vi "Compute Y's for equidistant Xn's.vi"(2 "Spline(T)":bool=TRUE, 3 "N":i16, 4 "Y":dbl[](array[numeric]) format="%.2e", 5 "X":dbl[](array[numeric]) format="%.2e") -> (0 "Yequi":dbl[](array[numeric]) format="%.2e", 1 "Xequi":dbl[](array[numeric]) format="%.2e")   [LabVIEW 2016]
doc: "Erzeugt zu einer XY-Meßkurve mit nicht \näquidistanten X-Werten eine zu \näquidistanten Werten. Die Größe N\nder neuen X- und Y-Arrays kann \ngrößer sein als die des Original X-Arrays.\nSpline gibt an, ob Spline- oder lineare\nInterpolation benutzt wird."
uses:
  <vilib>/Analysis/NI_AALPro.lvlib
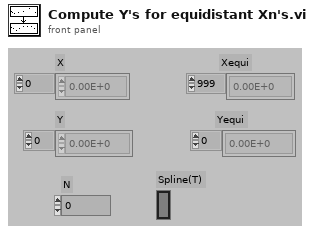
[diagram p1: front panel]
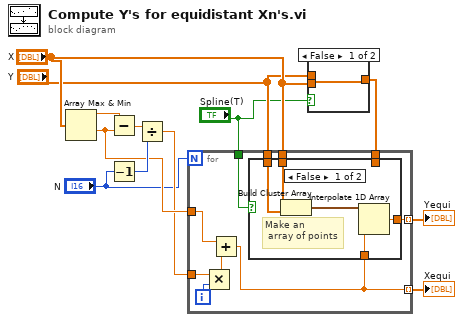
[diagram p0: block diagram]
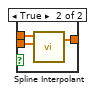
[diagram p2: hidden frame]
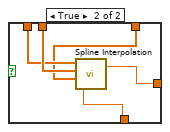
[diagram p3: hidden frame]
diagram:
  n1 = Array Max & Min(array="X") -> (max value=w12:dbl, min value=w9:dbl)  [unwired: 2 out]
  n2 = Subtract(x=w12, y=w9) -> (x-y=w11:dbl)
  n3 = Decrement(x="N") -> (x-1=w10:i16)
  n4 = Divide(x=w11, y=w10) -> (x/y=w8:dbl)
  n5 = case shown="False" "Spline(T)" {
    tunnel: [w13 w16] -> w5
    tunnel: "X" -> [w13 w15]
    tunnel: "Y" -> [_ w14]
    frame False {
    }
    frame True {
      n6 = call <vilib>:"Spline Interpolant.vi"("X"=w15, "Y"=w14) -> ("Interpolant"=w16:dbl[])  [unwired: 2 in, 1 out]
    }
  }
  n7 = for {
    N: "N" -> [_]
    tunnel: w9 -> [w26]
    tunnel: w8 -> [w23]
    tunnel: [w22] -> w7 mode=indexing
    tunnel: [w21] -> w6 mode=indexing
    tunnel: "X" -> [w20]
    tunnel: "Y" -> [w19]
    tunnel: w5 -> [w18]
    tunnel: "Spline(T)" -> [w17]
    i -> [w25]
    n8 = Multiply(x=w23, y=w25) -> (x*y=w24:dbl)
    n9 = Add(x=w26, y=w24) -> (x+y=w22:dbl)
    n10 = case shown="False" w17 {
      tunnel: [w31 w32] -> w21
      tunnel: w22 -> [w30 w33]
      tunnel: w20 -> [w29 w36]
      tunnel: w19 -> [w28 w35]
      tunnel: w18 -> [_ w34]
      frame False {
        # "Make an\n array of points"
        n11 = Build Cluster Array(w29, w28) -> (w27:cluster{dbl, dbl}[])
        n12 = Interpolate 1D Array(1:w30, 2:w27) -> (0:w31:dbl)
      }
      frame True {
        n13 = call <vilib>:"Spline Interpolation.vi"("x value"=w33, "Interpolant"=w34, "X"=w36, "Y"=w35) -> ("interpolation value"=w32:dbl)  [unwired: 1 out]
      }
    }
  }
  "Xequi" <- w7
  "Yequi" <- w6
